vi "Subvi clock.vi"() -> (2 "Output":bool)   [LabVIEW 2017]
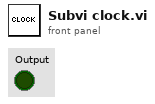
[diagram p1: front panel]
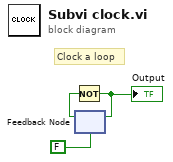
[diagram p0: block diagram]
diagram:
  # "Clock a loop"
  n1 = feedback #1(FALSE) -> (w3:bool)
  n2 = Not(x=w3) -> (.not. x?=w1:bool)
  "Output" <- w1
  n3 = feedback-in #1(w1) -> ()
